vi "Read Caller Enqueuer.vi"(11 "Interlock in":refnum<class "Interlock.lvclass">) -> (2 "Actor Framework:Message Enqueuer":refnum<class "Message Enqueuer.lvclass">, 3 "Interlock out":refnum<class "Interlock.lvclass">)   [LabVIEW 2015, in "Interlocks.lvlib" / "Interlock.lvclass"]
uses:
  Interlock.lvclass
  <vilib>/ActorFramework/Message Enqueuer/Message Enqueuer.lvclass
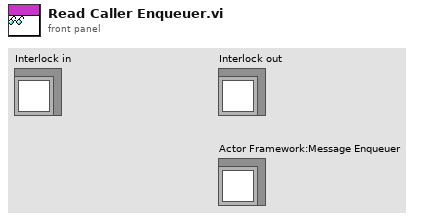
[diagram p1: front panel]
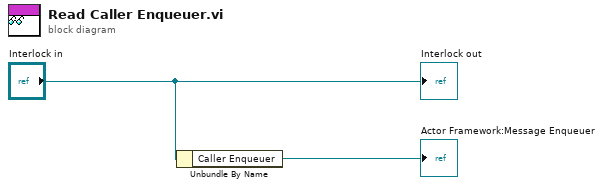
[diagram p0: block diagram]
diagram:
  n1 = Unbundle By Name("Interlock in") -> ("Caller Enqueuer"=→"Actor Framework:Message Enqueuer":refnum<class "Message Enqueuer.lvclass">)
  "Interlock out" <- "Interlock in"
